vi "AssertVIExecCore.vi"(0 "VI Reference In":refnum<vi>, 1 "Label":string, 3 "Assert Only? (F)":bool, 5 "Execution:State":T1(array[ring]), 11 "Error In":errorcluster, 12 "Assert Interval(10 ms)":u32=10, 13 "Timeout(5 sec)":dbl=5.0) -> (4 "VI Reference Out":refnum<vi>, 15 "Error Out":errorcluster)   [LabVIEW 2016, in "Drona.lvlib" / "AssertVI.lvlib"]
doc: "Asserts the state of controls.\n\nThe input control name is given as a string , incase of path, use delimiters inbetween the path."
uses:
  AssertVI.lvlib
  <vilib>/addons/_JKI Toolkits/Caraya/classes/Assert/Assert True.vi
  <vilib>/addons/_JKI Toolkits/Caraya/classes/Assert/Assert.lvclass
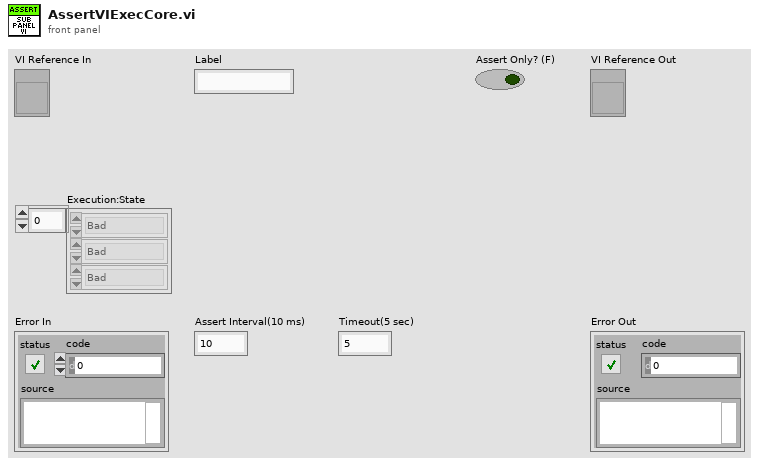
[diagram p1: front panel]
types:
  T1 = enum32{"Bad", "Idle", "Run top level", "Running"}[]
  T2 = enum32{"Bad", "Idle", "Run top level", "Running"}
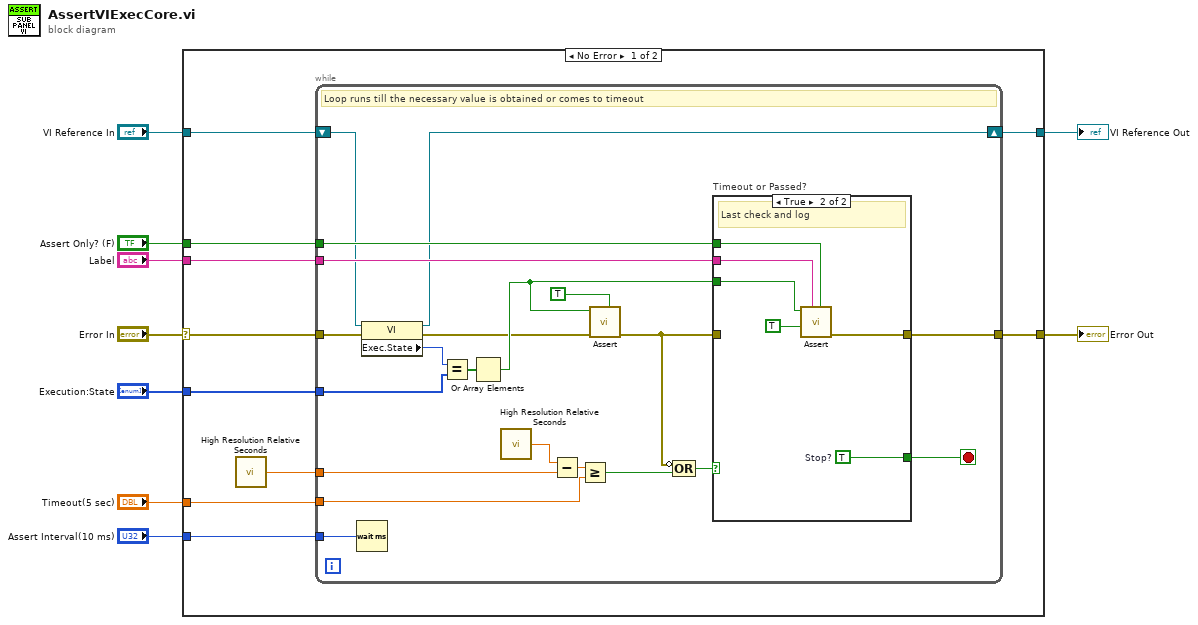
[diagram p0: block diagram]
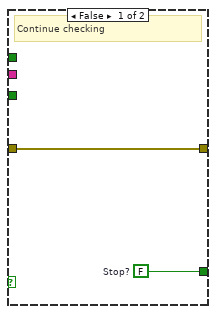
[diagram p2: hidden frame]
diagram:
  n1 = case shown="No Error" "Error In" {
    selector: "Error In" -> [w15 w50]
    tunnel: "Timeout(5 sec)" -> [w19 _]
    tunnel: [w18 w49] -> w8
    tunnel: [w10 w50] -> w7
    tunnel: "Assert Interval(10 ms)" -> [w17 _]
    tunnel: "Label" -> [w16 _]
    tunnel: "VI Reference In" -> [w14 w49]
    tunnel: "Assert Only? (F)" -> [w12 _]
    tunnel: "Execution:State" -> [w11 _]
    frame No Error {
      n2 = call <vilib>:"High Resolution Relative Seconds.vi"() -> ("relative seconds"=w13:dbl)
      n3 = while {
        tunnel: w19 -> [w39]
        tunnel: w13 -> [w40]
        tunnel: w15 -> [w35]
        tunnel: [w37] -> w10
        tunnel: w17 -> [w36]
        tunnel: w16 -> [w34]
        shift-right: [w20] -> w18
        shift-left: w14 -> [w21]
        tunnel: w12 -> [w33]
        tunnel: w11 -> [w32]
        stop <- w38 stop-if-true
        # "Loop runs till the necessary value is obtained or comes to timeout"
        n4 = Wait (ms)(milliseconds to wait=w36) -> ()  [unwired: 1 out]
        n5 = property class="VI"(reference=w21, error in=w35) -> (reference out=w20:refnum<vi>, error out=w22:errorcluster, "Exec.State"=w25:T2)
        n6 = Equal?(x=w25, y=w32) -> (x = y?=w24:bool[])
        n7 = Or Array Elements(Boolean array=w24) -> (logical OR=w23:bool)
        n8 = call <vilib>:"High Resolution Relative Seconds.vi"() -> ("relative seconds"=w31:dbl)
        n9 = Subtract(x=w31, y=w40) -> (x-y=w30:dbl)
        n10 = Greater Or Equal?(x=w30, y=w39) -> (x >= y?=w29:bool)
        n11 = call-poly <vilib>:"Assert.vi"("Assert Only? (F)"=TRUE, "error in (no error)"=w22, "True?"=w23) -> ("error out"=w28:errorcluster)  [unwired: 8 in]
        n12 = Compound Arithmetic op=OR(invert w28, w29) -> (w27:bool)
        n13 = case "Timeout or Passed?" shown="True" w27 {
          tunnel: w28 -> [w42 _]
          tunnel: w23 -> [_ w47]
          tunnel: w34 -> [_ w48]
          tunnel: [w42 w46] -> w37
          tunnel: [w41 w45] -> w38
          tunnel: w33 -> [_ w43]
          frame False {
            w41 = FALSE  # Stop?
            # "Continue checking"
          }
          frame True {
            w45 = TRUE  # Stop?
            # "Last check and log"
            n14 = call-poly <vilib>:"Assert.vi"("Assert Only? (F)"=w43, "Label"=w48, "Register with caller test (F)"=TRUE, "True?"=w47) -> ("error out"=w46:errorcluster)  [unwired: 7 in]
          }
        }
      }
    }
    frame Error {
    }
  }
  "Error Out" <- w7
  "VI Reference Out" <- w8
